vi "Subscribe.vi"(0 "mqtt in":refnum<class "MQTT Client.lvclass">, 5 "subscriptionInfo":T1[](array[typedef])=[{"Topic"="a/b", "QoS"=enum."At least once"}], 11 "error in (no error)":errorcluster) -> (4 "mqtt out":refnum<class "MQTT Client.lvclass">, 15 "error out":errorcluster)   [LabVIEW 2020, in "MQTT Client.lvclass"]
uses:
  MQTT Client.lvclass
  mqttTypedef/SubscribeData.ctl
  mqttTypedef/QosLevel.ctl
  mqttCmd/mqttCmdSubscribe/SubscribeMqttMsg.lvclass
  C:/Projects/Libraries/Gore SM 2020/mqtt-LabVIEW/src/class/mqtt/mqttCmd/BaseMqttMsg.lvclass
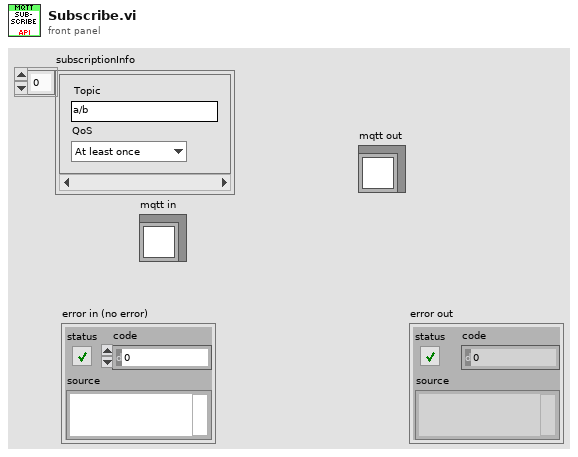
[diagram p1: front panel]
types:
  T1 = typedef "MQTT Client.lvclass/SubscribeData.ctl" = cluster{"Topic":string, "QoS":T2}
  T2 = typedef "MQTT Client.lvclass/QosLevel.ctl" = enum8{"At most once", "At least once", "Exactly once", "Reserved"}
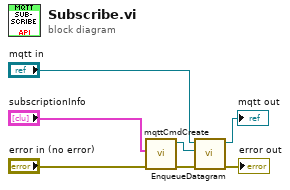
[diagram p0: block diagram]
diagram:
  n1 = call "mqttCmdCreate.vi"("error in (no error)"="error in (no error)", "subscriptionInfo"="subscriptionInfo") -> ("error out"=w4:errorcluster, "mqttCmdSubscribe out"=w3:refnum<class "SubscribeMqttMsg.lvclass">)  [unwired: 8 in]
  n2 = call "EnqueueDatagram.vi"("error in (no error)"=w4, "mqttCmd"=w3, "mqtt in"="mqtt in") -> ("error out"=→"error out":errorcluster, "mqtt out"=→"mqtt out":refnum<class "MQTT Client.lvclass">)  [unwired: 7 in]
